vi "Draw Circles.vi"(10 "Print Ouptut":string, 11 "Refnum in":T1) -> (3 "Refnum out":T1)   [LabVIEW 2020]
uses:
  <vilib>/vision/Image Controls.llb/IMAQ Image.ctl
  <vilib>/regexp/Match Regular Expression.xnode
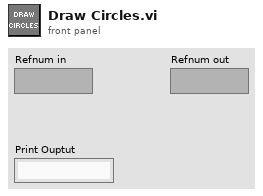
[diagram p1: front panel]
types:
  T1 = typedef "IMAQ Image.ctl" = refnum<image>
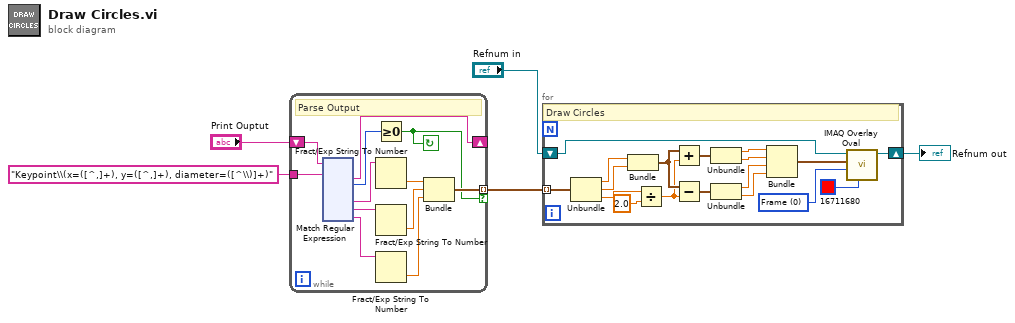
[diagram p0: block diagram]
diagram:
  n1 = while {
    shift-right: [w16] -> _
    shift-left: "Print Ouptut" -> [w17]
    tunnel: "Keypoint\\(x=([^,]+), y=([^,]+), diameter=([^\\)]+)" ("regular expression") -> [w11]
    tunnel: [w7] -> w3 mode=indexing if=w6
    stop <- w6 continue-if-true
    # "Parse Output"
    n2 = xnode "Match Regular Expression"("input string"=w17, "regular expression"=w11) -> ("after match"=w16:string, "offset past match"=w15:i32, "submatch 1"=w14:string, "submatch 2"=w13:string, "submatch 3"=w12:string)  [unwired: 4 in, 3 out]
    n3 = Greater Or Equal To 0?(x=w15) -> (x >= 0?=w6:bool)
    n4 = Fract/Exp String To Number(string=w14) -> (number=w10:dbl)  [unwired: 3 in, 1 out]
    n5 = Fract/Exp String To Number(string=w13) -> (number=w9:dbl)  [unwired: 3 in, 1 out]
    n6 = Fract/Exp String To Number(string=w12) -> (number=w8:dbl)  [unwired: 3 in, 1 out]
    n7 = Bundle(w10, w9, w8) -> (w7:cluster{dbl, dbl, dbl})  [unwired: 1 in]
  }
  n8 = for {
    tunnel: w3 -> [w152] mode=indexing
    shift-right: [w150] -> w5
    shift-left: "Refnum in" -> [w153]
    w136 = u32 0 items=["Frame", "Fill"] ("Drawing Mode (Frame)")
    # "Draw Circles"
    n9 = Unbundle(w152) -> (w147:dbl, w146:dbl, w149:dbl)
    n10 = Bundle(w147, w146) -> (w145:cluster{dbl, dbl})  [unwired: 1 in]
    n11 = Divide(x=w149, y=2.0) -> (x/y=w144:dbl)
    n12 = Add(x=w145, y=w144) -> (x+y=w143:cluster{dbl, dbl})
    n13 = Subtract(x=w145, y=w144) -> (x-y=w142:cluster{dbl, dbl})
    n14 = Unbundle(w143) -> (w141:dbl, w140:dbl)
    n15 = Unbundle(w142) -> (w139:dbl, w138:dbl)
    n16 = Bundle(w141, w140, w139, w138) -> (w137:cluster{dbl, dbl, dbl, dbl})  [unwired: 1 in]
    n17 = call "IMAQ Overlay Oval"("Color"=u32 16711680, "Drawing Mode (Frame)"=w136, "Bounding Rectangle"=w137, "Image"=w153) -> ("Image Out"=w150:T1)  [unwired: 6 in, 1 out]
  }
  "Refnum out" <- w5
